vi "FPGA-DataIn.vi"(0 "Nr of Analog Inputs":i16=2) -> (1 "AnalogIn0":u16, 2 "AnalogIn1":u16, 3 "AnalogIn2":u16, 4 "AnalogIn3":u16)   [LabVIEW 2020]
uses:
  <vilib>/rvi/Emulation/niFpgaGetClockAttributes.vi
  <vilib>/rvi/Emulation/niFpgaSctlEmulationGetInTimedLoop.vi
  <vilib>/rvi/Emulation/niFpgaEmulationReportErrorSimple.vi
  <vilib>/rvi/eio/common/nirviEmuTemplateMethod_errors.vi
  <vilib>/rvi/Emulation/niFpgaCriticalErrorInLSC.vi
  <vilib>/eio/EIONode/EIONode.xnode
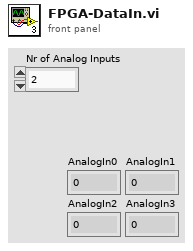
[diagram p1: front panel]
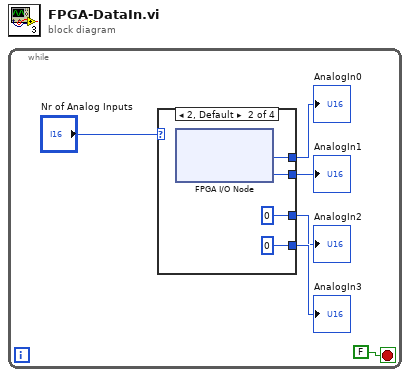
[diagram p0: block diagram]
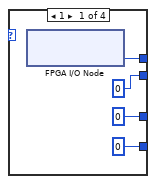
[diagram p2: hidden frame]
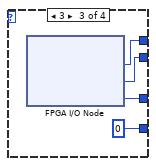
[diagram p3: hidden frame]
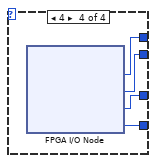
[diagram p4: hidden frame]
diagram:
  n1 = while {
    stop <- FALSE stop-if-true
    n2 = case shown="2, Default" "Nr of Analog Inputs" {
      tunnel: [u16 0 ("AnalogIn3") u16 0 ("AnalogIn3") u16 0 ("AnalogIn3") w22] -> w5
      tunnel: [u16 0 ("AnalogIn2") u16 0 ("AnalogIn2") w18 w21] -> w4
      tunnel: [u16 0 ("AnalogIn1") w14 w17 w20] -> w3
      tunnel: [w10 w13 w16 w19] -> w2
      frame 1 {
        n3 = xnode "FPGA I/O Node"() -> ("AnalogIn0"=w10:u16)  [unwired: 1 in, 1 out]
      }
      frame 2, Default {
        n4 = xnode "FPGA I/O Node"() -> ("AnalogIn0"=w13:u16, "AnalogIn1"=w14:u16)  [unwired: 2 in, 2 out]
      }
      frame 3 {
        n5 = xnode "FPGA I/O Node"() -> ("AnalogIn0"=w16:u16, "AnalogIn1"=w17:u16, "AnalogIn2"=w18:u16)  [unwired: 3 in, 3 out]
      }
      frame 4 {
        n6 = xnode "FPGA I/O Node"() -> ("AnalogIn0"=w19:u16, "AnalogIn1"=w20:u16, "AnalogIn2"=w21:u16, "AnalogIn3"=w22:u16)  [unwired: 4 in, 4 out]
      }
    }
    "AnalogIn0" <- w2
    "AnalogIn1" <- w3
    "AnalogIn2" <- w4
    "AnalogIn3" <- w5
  }
